vi "Actor Core.vi"(8 "error in":errorcluster, 11 "DAQ Device in":refnum<class "DAQ Device.lvclass">) -> (0 "error out":errorcluster, 3 "Actor out":refnum<class "Actor.lvclass">)   [LabVIEW 2014, in "DAQ Device.lvclass"]
doc: "(<B>Filename</B>: Actor Framework.lvlib:Actor.lvclass:Actor Core.vi)\n\nReceives messages to the actor, reacts to them, and initiates any error handling that may shut the actor down.\n\nDescendant classes may override this VI to append parallel tasks for the actor to complete while it handles messages. Overrides use the Call Parent Method node."
uses:
  DAQ Device.lvclass
  <vilib>/ActorFramework/Actor/Actor.lvclass
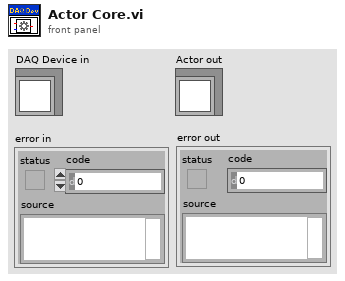
[diagram p1: front panel]
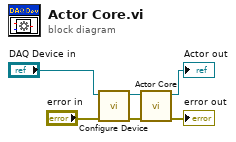
[diagram p0: block diagram]
diagram:
  n1 = call-dynamic "Configure Device.vi"("error in"="error in", "DAQ Device in"="DAQ Device in") -> ("error out"=w2:errorcluster, "DAQ Device out"=w1:refnum<class "DAQ Device.lvclass">)  [unwired: 8 in]
  n2 = call-parent "Actor Core.vi"("error in"=w2, "Actor in"=w1) -> ("error out"=→"error out":errorcluster, "Actor out"=→"Actor out":refnum<class "Actor.lvclass">)  [unwired: 8 in]
